vi "RSZVB Set Coherent Signal State.vi"(7 "Coherent Signal (F: Off)":bool, 8 "error in (no error)":errorcluster {"code" format="%.0x"}, 9 "Port (1)":i32=1, 10 "Channel (1)":i32=1, 11 "VISA session":refnum<visa-resource-name>) -> (0 "error out":errorcluster {"code" format="%.0x"}, 3 "dup VISA session":refnum<visa-resource-name>)   [LabVIEW 2011]
doc: "This VI qualifies whether the signal at port no. <Pt> is a coherent or a non-coherent signal.\n\nNote(s):\n\n(1) This VI is not available for R&S ZVB instrument.\n\nRemote-control command(s):\nSOURce<Ch>:CMODe:PORT<Pt>[:STATe] ON | OFF"
uses:
  _utility/RSZVB Global Data.vi
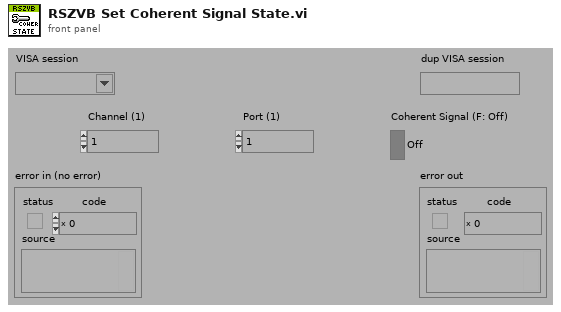
[diagram p1: front panel]
types:
  T1 = cluster{"Error Checking (T: On)":bool, "Installed Options":string[], "Data Valid?":bool, "Ports":i32, "Model":string[], "Option Checking (T: On)":bool}[]
  T2 = cluster{"Error Checking (T: On)":bool, "Installed Options":string[], "Data Valid?":bool, "Ports":i32, "Model":string[], "Option Checking (T: On)":bool}
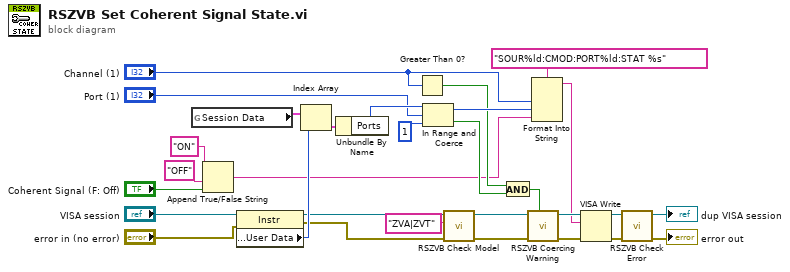
[diagram p0: block diagram]
diagram:
  n1 = global read "RSZVB Global Data.vi" "Session Data"() -> (w25:T1)
  n2 = Append True/False String(1:"Coherent Signal (F: Off)", 2:"OFF" ("false string"), 3:"ON" ("true string")) -> (0:w6:string)  [unwired: 1 in]
  n3 = property class="Instr"(reference="VISA session", error in="error in (no error)") -> (reference out=w2:refnum<visa-resource-name>, error out=w1:errorcluster, "General Settings:User Data"=w27:u32)
  n4 = Index Array(array=w25, index=w27) -> (element=w24:T2)
  n5 = Unbundle By Name(w24) -> ("Ports"=w28:i32)
  n6 = Greater Than 0?(x="Channel (1)") -> (x > 0?=w7:bool)
  n7 = In Range and Coerce(upper limit=w28, x="Port (1)", lower limit=1) -> (coerced(x)=w29:i32, In Range?=w8:bool)
  n8 = call "RSZVB Check Model.vi"("error in (no error)"=w1, "Model"="ZVA|ZVT", "VISA session"=w2) -> ("error out"=w3:errorcluster, "dup VISA session"=w4:refnum<visa-resource-name>)  [unwired: 7 in]
  n9 = And(x=w7, y=w8) -> (x .and. y?=w30:bool)
  n10 = call "RSZVB Coercing Warning.vi"("In Range?"=w30, "error in (no error)"=w3, "VISA session"=w4) -> ("error out"=w21:errorcluster, "dup VISA session"=w22:refnum<visa-resource-name>)  [unwired: 7 in]
  n11 = Format Into String(format string="SOUR%ld:CMOD:PORT%ld:STAT %s", "Channel (1)", w29, w6) -> (resulting string=w20:string)  [unwired: 2 in, 1 out]
  n12 = VISA Write(VISA resource name=w22, write buffer=w20, error in (no error)=w21) -> (VISA resource name out=w19:refnum<visa-resource-name>, error out=w18:errorcluster)  [unwired: 1 out]
  n13 = call "RSZVB Check Error.vi"("error in (no error)"=w18, "VISA session"=w19) -> ("error out"=→"error out":errorcluster, "dup VISA session"=→"dup VISA session":refnum<visa-resource-name>)  [unwired: 8 in]
